vi "tcs_putSample_kernelPointingLog.vi"(8 "error in (no error)":errorcluster, 11 "kernel_PointingLog_Ctl":T1={"Aux[3]"=[0.0, 0.0, 0.0], "Casspa"=0.0, "Dec"=0.0, "Fl"=0.0, "Humid"=0.0, "Marked"=0, "Pitch"=0.0, "Press"=0.0, "Ra"=0.0, "Rcorr"=0.0, "Roll"=0.0, "Temp"=0.0, "Tlr"=0.0, "Wavel"=0.0, "Xr"=0.0, "Yr"=0.0}) -> (0 "error out":errorcluster, 2 "function return":i32, 3 "kernel_PointingLog_Ctl out":T1)   [LabVIEW 2016, in "SALLV_tcs.lvlib"]
doc: "int tcs_shm_putSample_kernel_PointingLogLV(tcs_kernel_PointingLogLV *kernel_PointingLog_Ctl );"
uses:
  SALLV_tcs.lvlib
  DataTypes/kernel_PointingLog.ctl
  SALLV_tcs.so
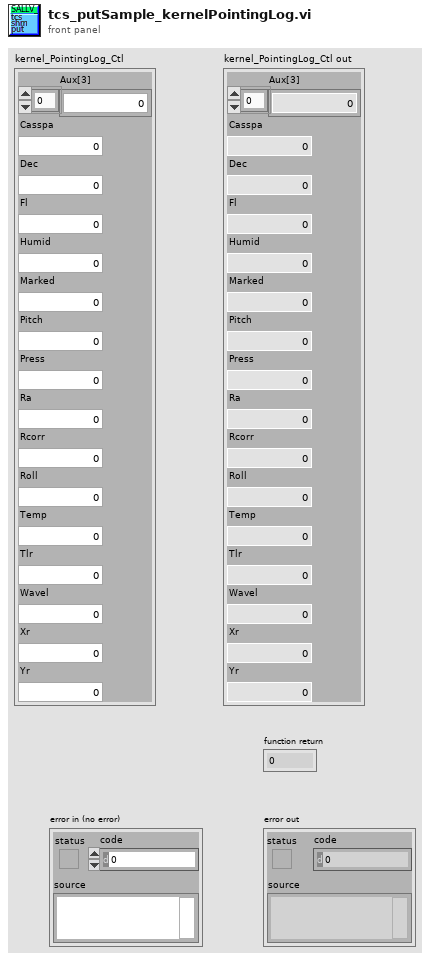
[diagram p1: front panel]
types:
  T1 = typedef "SALLV_tcs.lvlib/kernel_PointingLog.ctl" = cluster{"Aux[3]":sgl[], "Casspa":sgl, "Dec":sgl, "Fl":sgl, "Humid":sgl, "Marked":i32, "Pitch":sgl, "Press":sgl, "Ra":sgl, "Rcorr":sgl, "Roll":sgl, "Temp":sgl, "Tlr":sgl, "Wavel":sgl, "Xr":sgl, "Yr":sgl}
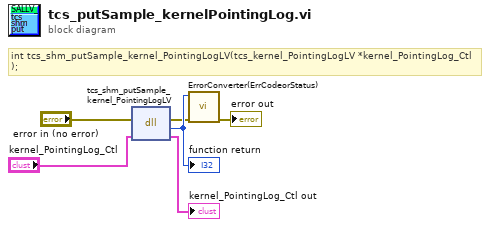
[diagram p0: block diagram]
diagram:
  # "int tcs_shm_putSample_kernel_PointingLogLV(tcs_kernel_PointingLogLV *kernel_PointingLog_Ctl );"
  n1 = dll-call lib="home/andres/Desktop/SALLV_tcs/SALLV_tcs.*" fn="tcs_shm_putSample_kernel_PointingLogLV"(error in="error in (no error)", "kernel_PointingLog_Ctl"="kernel_PointingLog_Ctl") -> (error out=w2:errorcluster, w6:i32, "kernel_PointingLog_Ctl"=→"kernel_PointingLog_Ctl out":T1)  [unwired: 2 in, 1 out]
  "function return" <- w6
  n2 = call "ErrorConverter(ErrCodeorStatus).vi"("error in (no error)"=w2, "error code"=w6) -> ("error out"=→"error out":errorcluster)  [unwired: 9 in]
